vi "Stop acquisition.vi"(8 "error in (no error)":errorcluster, 10 "buffer ref":i32, 11 "camera handle in":i16) -> (0 "error out":errorcluster, 3 "camera handle out":i16)   [LabVIEW 2012]
uses:
  Visual Studio/Cascade wrapper/Release/Cascade wrapper.dll
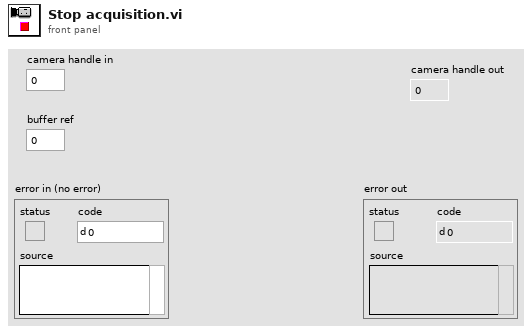
[diagram p1: front panel]
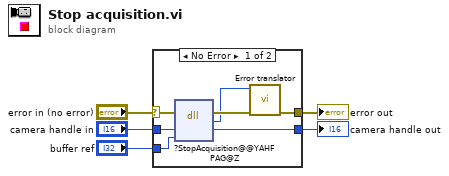
[diagram p0: block diagram]
diagram:
  n1 = case shown="No Error" "error in (no error)" {
    selector: "error in (no error)" -> [w12 w14]
    tunnel: [w10 w14] -> w4
    tunnel: "camera handle in" -> [w8 w13]
    tunnel: [w7 w13] -> w2
    tunnel: "buffer ref" -> [w6 _]
    frame No Error {
      n2 = dll-call lib="C:/moroder/Cascade wrapper/Visual Studio/Cascade wrapper/Release/Cascade wrapper.dll" fn="?StopAcquisition@@YAHFPAG@Z"(error in=w12, "camera handle"=w8, "buffer ref"=w6) -> (error out=w11:errorcluster, "error"=w9:i32, "camera handle"=w7:i16)  [unwired: 3 in, 1 out]
      n3 = call "Error translator.vi"("error in (no error)"=w11, "error code"=w9) -> ("error out"=w10:errorcluster)  [unwired: 9 in]
    }
    frame Error {
    }
  }
  "error out" <- w4
  "camera handle out" <- w2
